vi "Write Name.vi"(8 "error in (no error)":errorcluster, 10 "Name":string, 11 "Event Sink in":refnum<class "Event Sink.lvclass">) -> (0 "error out":errorcluster, 3 "Event Sink out":refnum<class "Event Sink.lvclass">)   [LabVIEW 2016, in "Event Source.lvlib" / "Event Sink.lvclass"]
uses:
  Event Sink.lvclass
  Event Sink.lvclass/Event Sink.ctl
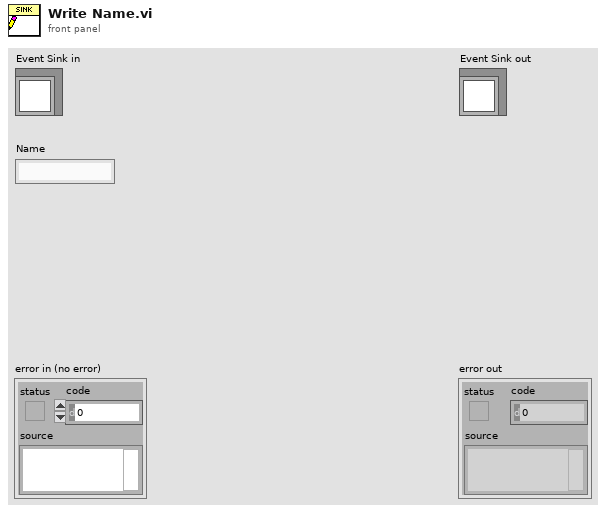
[diagram p1: front panel]
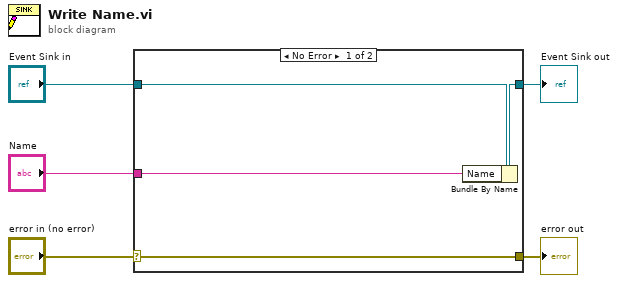
[diagram p0: block diagram]
diagram:
  n1 = case shown="No Error" "error in (no error)" {
    selector: "error in (no error)" -> [w9 w10]
    tunnel: [w9 w10] -> w4
    tunnel: [w7 w11] -> w2
    tunnel: "Event Sink in" -> [w8 w11]
    tunnel: "Name" -> [w6 _]
    frame No Error {
      n2 = Bundle By Name(cluster=w8, "Name"=w6) -> (w7:refnum<class "Event Sink.lvclass">)
    }
    frame Error {
    }
  }
  "error out" <- w4
  "Event Sink out" <- w2
